vi "CRYInit Project Editor.vi"(6 "Pane 3":refnum<vi>, 8 "Splitter 2":refnum<vi>, 9 "Pane 2":refnum<vi>, 10 "Splitter 1":refnum<vi>, 11 "Pane 1":refnum<vi>) -> ()   [LabVIEW 2013]
uses:
  <vilib>/Utility/miscctls.llb/LVPositionTypeDef.ctl
  CRYProject Editor Global.vi
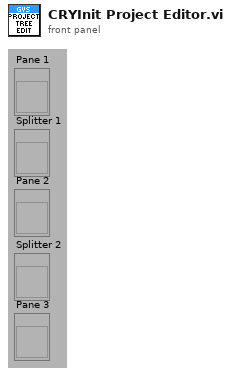
[diagram p1: front panel]
types:
  T1 = typedef "LVPositionTypeDef.ctl" = cluster{"Left":i32, "Top":i32}
  T2 = typedef "LVRectTypeDef.ctl" = cluster{"Left":i16, "Top":i16, "Right":i16, "Bottom":i16}
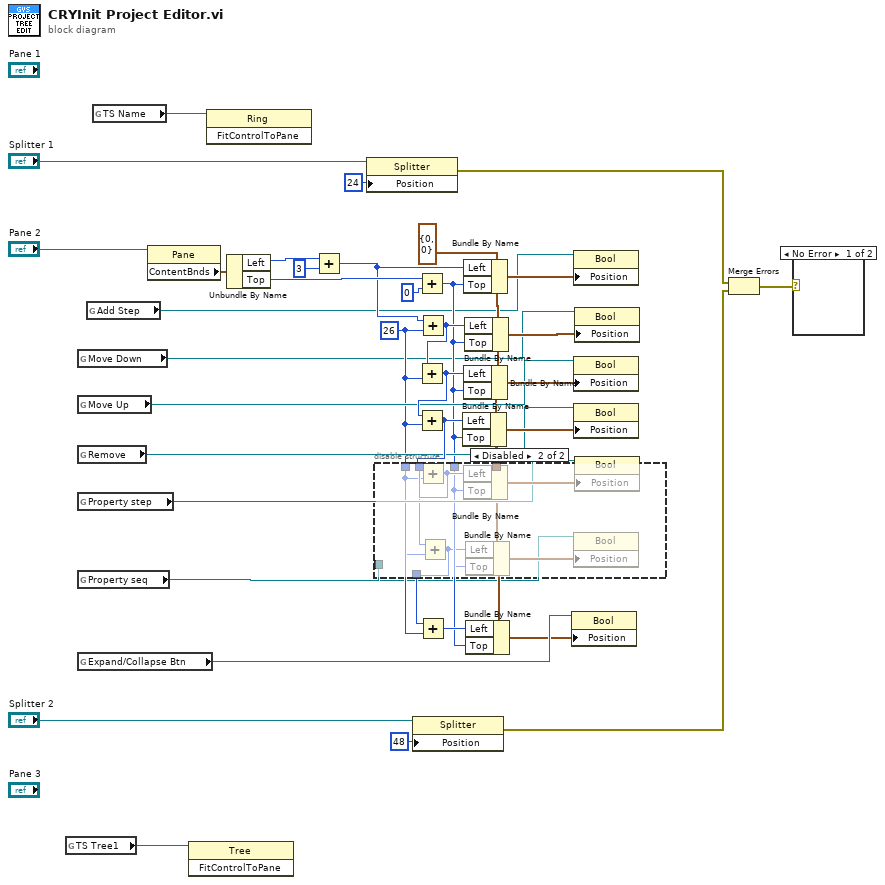
[diagram p0: block diagram]
diagram:
  w5 = i16 26 ("y")
  w7 = T1 {"Left"=0, "Top"=0} ("Position")
  n1 = global read "CRYProject Editor Global.vi" "TS Tree1"() -> (w19:refnum<vi>)
  n2 = global read "CRYProject Editor Global.vi" "Move Down"() -> (w1:refnum<vi>)
  n3 = global read "CRYProject Editor Global.vi" "Move Up"() -> (w23:refnum<vi>)
  n4 = global read "CRYProject Editor Global.vi" "Remove"() -> (w22:refnum<vi>)
  n5 = global read "CRYProject Editor Global.vi" "Property step"() -> (w21:refnum<vi>)
  n6 = global read "CRYProject Editor Global.vi" "Property seq"() -> (w20:refnum<vi>)
  n7 = global read "CRYProject Editor Global.vi" "Expand/Collapse Btn"() -> (w13:refnum<vi>)
  n8 = global read "CRYProject Editor Global.vi" "Add Step"() -> (w2:refnum<vi>)
  n9 = global read "CRYProject Editor Global.vi" "TS Name"() -> (w16:refnum<vi>)
  n10 = property class="Pane"(reference="Pane 2") -> ("ContentBnds"=w38:T2)  [unwired: 1 in, 2 out]
  n11 = invoke class="Tree" method="FitControlToPane"(reference=w19) -> ()  [unwired: 2 in, 3 out]
  n12 = invoke class="Ring" method="FitControlToPane"(reference=w16) -> ()  [unwired: 2 in, 3 out]
  n13 = Unbundle By Name(w38) -> ("Left"=w29:i16, "Top"=w32:i16)
  n14 = Add(x=w29, y=i16 3) -> (x+y=w6:i16)
  n15 = property on="Property Node" class="Splitter"(reference="Splitter 1", "Position"=24 ("Splitter Position")) -> (error out=w11:errorcluster)  [unwired: 1 in, 1 out]
  n16 = property on="Property Node" class="Splitter"(reference="Splitter 2", "Position"=48 ("Splitter Position")) -> (error out=w10:errorcluster)  [unwired: 1 in, 1 out]
  n17 = Add(x=w32, y=i16 0) -> (x+y=w3:i16)
  n18 = Add(x=w6, y=w5) -> (x+y=w4:i16)
  n19 = Add(x=w4, y=w5) -> (x+y=w28:i16)
  n20 = Add(x=w28, y=w5) -> (x+y=w27:i16)
  n21 = Add(x=w27, y=w5) -> (x+y=w26:i16)
  n22 = disable-structure shown="Disabled" {
    disable-tunnel: w26 -> [w39 w45]
    disable-tunnel: w20 -> [_ w44]
    disable-tunnel: [w39 w43] -> w14
    disable-tunnel: w5 -> [_ w42]
    disable-tunnel: w3 -> [_ w41]
    disable-tunnel: w7 -> [_ w40]
    frame Enabled {
    }
    frame Disabled {
      n23 = Add(x=w45, y=w42) -> (x+y=w43:i16)
      n24 = Bundle By Name(cluster=w40, "Left"=w43, "Top"=w41) -> (w46:T1)
      n25 = property class="Bool"(reference=w44, "Position"=w46) -> ()  [unwired: 1 in, 2 out]
    }
  }
  n26 = Add(x=w14, y=w5) -> (x+y=w15:i16)
  n27 = Bundle By Name(cluster=w7, "Left"=w27, "Top"=w3) -> (w34:T1)
  n28 = Bundle By Name(cluster=w7, "Left"=w6, "Top"=w3) -> (w37:T1)
  n29 = Bundle By Name(cluster=w7, "Left"=w28, "Top"=w3) -> (w35:T1)
  n30 = Bundle By Name(cluster=w7, "Left"=w26, "Top"=w3) -> (w31:T1)
  n31 = Bundle By Name(cluster=w7, "Left"=w4, "Top"=w3) -> (w8:T1)
  n32 = Bundle By Name(cluster=w7, "Left"=w15, "Top"=w3) -> (w12:T1)
  n33 = property class="Bool"(reference=w13, "Position"=w12) -> ()  [unwired: 1 in, 2 out]
  n34 = property on="Property Node" class="Bool"(reference=w2, "Position"=w37) -> ()  [unwired: 1 in, 2 out]
  n35 = property on="Property Node" class="Bool"(reference=w23, "Position"=w35) -> ()  [unwired: 1 in, 2 out]
  n36 = property on="Property Node" class="Bool"(reference=w22, "Position"=w34) -> ()  [unwired: 1 in, 2 out]
  n37 = property on="Property Node" class="Bool"(reference=w1, "Position"=w8) -> ()  [unwired: 1 in, 2 out]
  n38 = property on="Property Node" class="Bool"(reference=w21, "Position"=w31) -> ()  [unwired: 1 in, 2 out]
  n39 = Merge Errors(w11, w10) -> (w9:errorcluster)
  n40 = case shown="No Error" w9 {
    frame No Error {
    }
    frame Error {
    }
  }
